vi "Configure PKCE.vi"(7 "Use PKCE? (T)":bool=TRUE, 8 "error in":errorcluster, 11 "Oauth2 in":refnum<class "Oauth2.lvclass">) -> (0 "error out":errorcluster, 3 "Oauth2":refnum<class "Oauth2.lvclass">)   [LabVIEW 2013, in "Oauth2.lvclass"]
uses:
  Oauth2.lvclass
  OAuthToken/OAuth2 Token Element -- enum.ctl
  Oauth2.lvclass/Oauth2.ctl
  <vilib>/LabVIEW Open Source Project/OpenSerializer.Base64/Serializer.Base64.lvclass/Serializer.Base64.ctl
  Utilities/SHA-256/Compute SHA256 (byte array).vi
  <vilib>/LabVIEW Open Source Project/OpenSerializer.Base64/Base64url_CharSet.vi
  <vilib>/LabVIEW Open Source Project/OpenSerializer.Base64/Write charset.vi
  Utilities/SHA-256/Get Block Size.vi
  Utilities/SHA-256/generators/SHA-256.vi
  Utilities/SHA-256/Pad.vi
  Utilities/SHA-256/Append Block.vi
  Utilities/SHA-256/Get Digest.vi
  Utilities/SHA-256/Reset.vi
  <vilib>/LabVIEW Open Source Project/OpenSerializer.Base64/Encode.vi
  <vilib>/LabVIEW Open Source Project/OpenSerializer.Base64/Serializer.Base64.lvclass
  OAuthToken/OAuthAccessToken.lvclass
  <vilib>/LabVIEW Open Source Project/Unicity/RandomStringGenerator/RandomStringGenerator.lvclass
  Utilities/SHA-256/NI_SHA-256(2013).lvlib
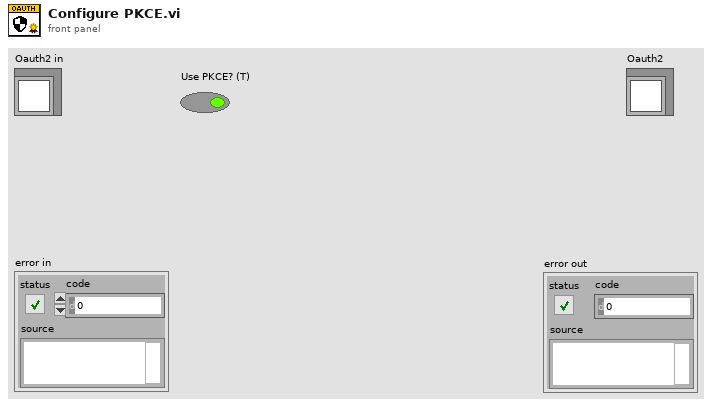
[diagram p1: front panel]
types:
  T1 = typedef "OAuthAccessToken.lvclass/OAuth2 Token Element -- enum.ctl" = enum16{"client_id", "client_secret", "response_type", "scope", "redirect_uri", "error", "error_description", "error_uri", "grant_type", "code", "access_token", "token_type", "expires_in", "username", "password", "refresh_token", "code_challenge", "code_challenge_method", "reverse_proxy_uri", "endpoint element"}
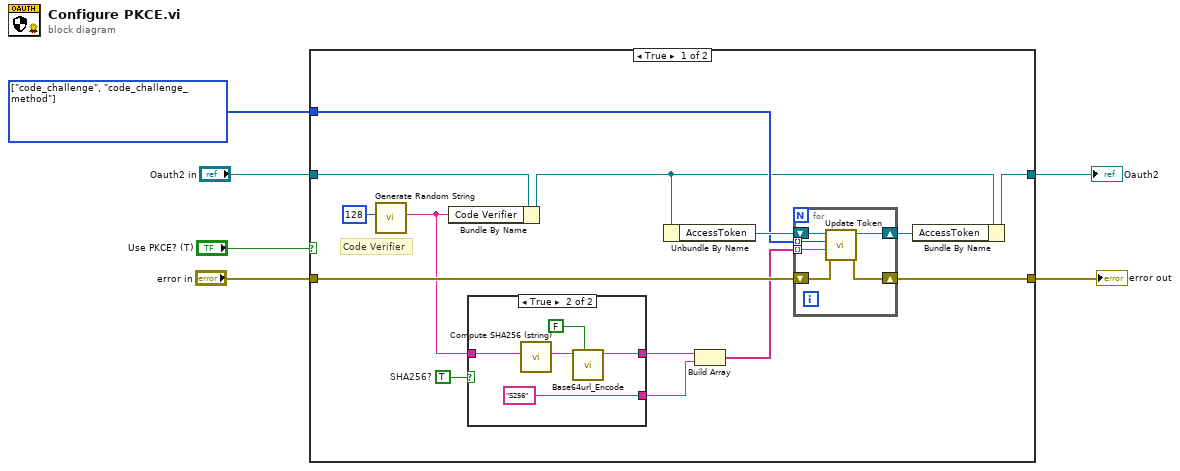
[diagram p0: block diagram]
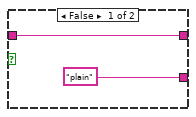
[diagram p2: hidden frame]
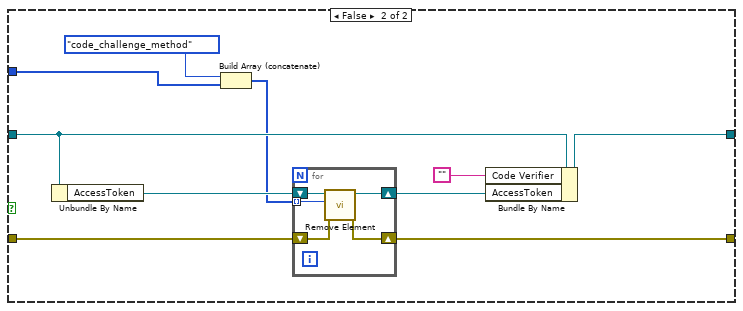
[diagram p3: hidden frame]
diagram:
  w5 = T1[] [enum."code_challenge", enum."code_challenge_method"] items=["client_id", "client_secret", "response_type", "scope", "redirect_uri", "error", "error_description", "error_uri", "grant_type", "code", "access_token", "token_type", "expires_in", "username", "password", "refresh_token", "code_challenge", "code_challenge_method", "reverse_proxy_uri", "endpoint element"]
  n1 = case shown="True" "Use PKCE? (T)" {
    tunnel: [w19 w42] -> w6
    tunnel: w5 -> [w17 w35]
    tunnel: [w16 w40] -> w4
    tunnel: "Oauth2 in" -> [w12 w39]
    tunnel: "error in" -> [w15 w38]
    frame True {
      w9 = TRUE  # SHA256?
      # "Code Verifier"
      n2 = call <vilib>:"Generate Random String.vi"("String Length (32)"=u32 128) -> ("Random String"=w10:string)  [unwired: 10 in]
      n3 = Bundle By Name(cluster=w12, "Code Verifier"=w10) -> (w11:refnum<class "Oauth2.lvclass">)
      n4 = case shown="True" w9 {
        tunnel: [w22 w24] -> w7
        tunnel: w10 -> [w22 w26]
        tunnel: ["plain" ("argument") "S256" ("argument")] -> w8
        frame False {
        }
        frame True {
          n5 = call "Compute SHA256 (string).vi"("String"=w26) -> ("hash"=w25:string)  [unwired: 10 in]
          n6 = call <vilib>:"Base64url_Encode.vi"("Padded (T)"=FALSE, "String"=w25) -> ("Encoded String"=w24:string)  [unwired: 8 in, 1 out]
        }
      }
      n7 = Unbundle By Name(w11) -> ("AccessToken"=w20:refnum<class "OAuthAccessToken.lvclass">)
      n8 = Build Array(w7, w8) -> (w13:string[])
      n9 = for {
        tunnel: w13 -> [w32] mode=indexing
        shift-right: [w31] -> w18
        shift-left: w20 -> [w33]
        tunnel: w17 -> [w30] mode=indexing
        shift-right: [w28] -> w16
        shift-left: w15 -> [w29]
        n10 = call "Update Token.vi"("error in (no error)"=w29, "Value"=w32, "Token element"=w30, "OAuthAccessToken in"=w33) -> ("error out"=w28:errorcluster, "OAuthAccessToken out"=w31:refnum<class "OAuthAccessToken.lvclass">)  [unwired: 6 in]
      }
      n11 = Bundle By Name(cluster=w11, "AccessToken"=w18) -> (w19:refnum<class "Oauth2.lvclass">)
    }
    frame False {
      n12 = Unbundle By Name(w39) -> ("AccessToken"=w43:refnum<class "OAuthAccessToken.lvclass">)
      n13 = Build Array (concatenate)(OAuth2_Token_Element_--_enum."code_challenge_method" ("Token element"), w35) -> (w34:T1[])
      n14 = for {
        shift-right: [w47] -> w41
        shift-left: w43 -> [w48]
        tunnel: w34 -> [w44] mode=indexing
        shift-right: [w46] -> w40
        shift-left: w38 -> [w45]
        n15 = call "Remove Element.vi"("error in (no error)"=w45, "Token element"=w44, "OAuthAccessToken in"=w48) -> ("error out"=w46:errorcluster, "OAuthAccessToken out"=w47:refnum<class "OAuthAccessToken.lvclass">)  [unwired: 6 in, 1 out]
      }
      n16 = Bundle By Name(cluster=w39, "Code Verifier"="", "AccessToken"=w41) -> (w42:refnum<class "Oauth2.lvclass">)
    }
  }
  "Oauth2" <- w6
  "error out" <- w4
